vi "HEWH Get Rates.vi"(0 "Software Elapsed Time":T1 format="%<%H:%M:%S>t", 1 "Test Type - Rate":string(combo)="Rate", 5 "ANSI Rate in":T3, 9 "Gas Measurment Data":T2, 11 "error in (no error)":errorcluster, 12 "Gross Heating Value, Vol (Real, Dry)":dbl=1000.0 min=900.0 max=2600.0 step=1.0, 13 "CO CO2 Data Array":string[][](array[string])) -> (3 "ANSI Display 1":string, 4 "Rate Outputs":string[][](array[string]), 6 "Test Complete":bool, 10 "ANSI Rate out":T3, 14 "Raw Timer Output":T1 format="%<%H:%M:%S>t", 15 "error out":errorcluster)   [LabVIEW 2019]
uses:
  Range/Type Definitions/RANGE ANSI Rate.ctl
  Utility/Custom Pallet Controls/Custom Pallet Timer.ctl
  Drivers/Alicat Gas Meter Driver/Sub-VIs/Data Cluster.ctl
panel:
  # "Totalizer Timer"
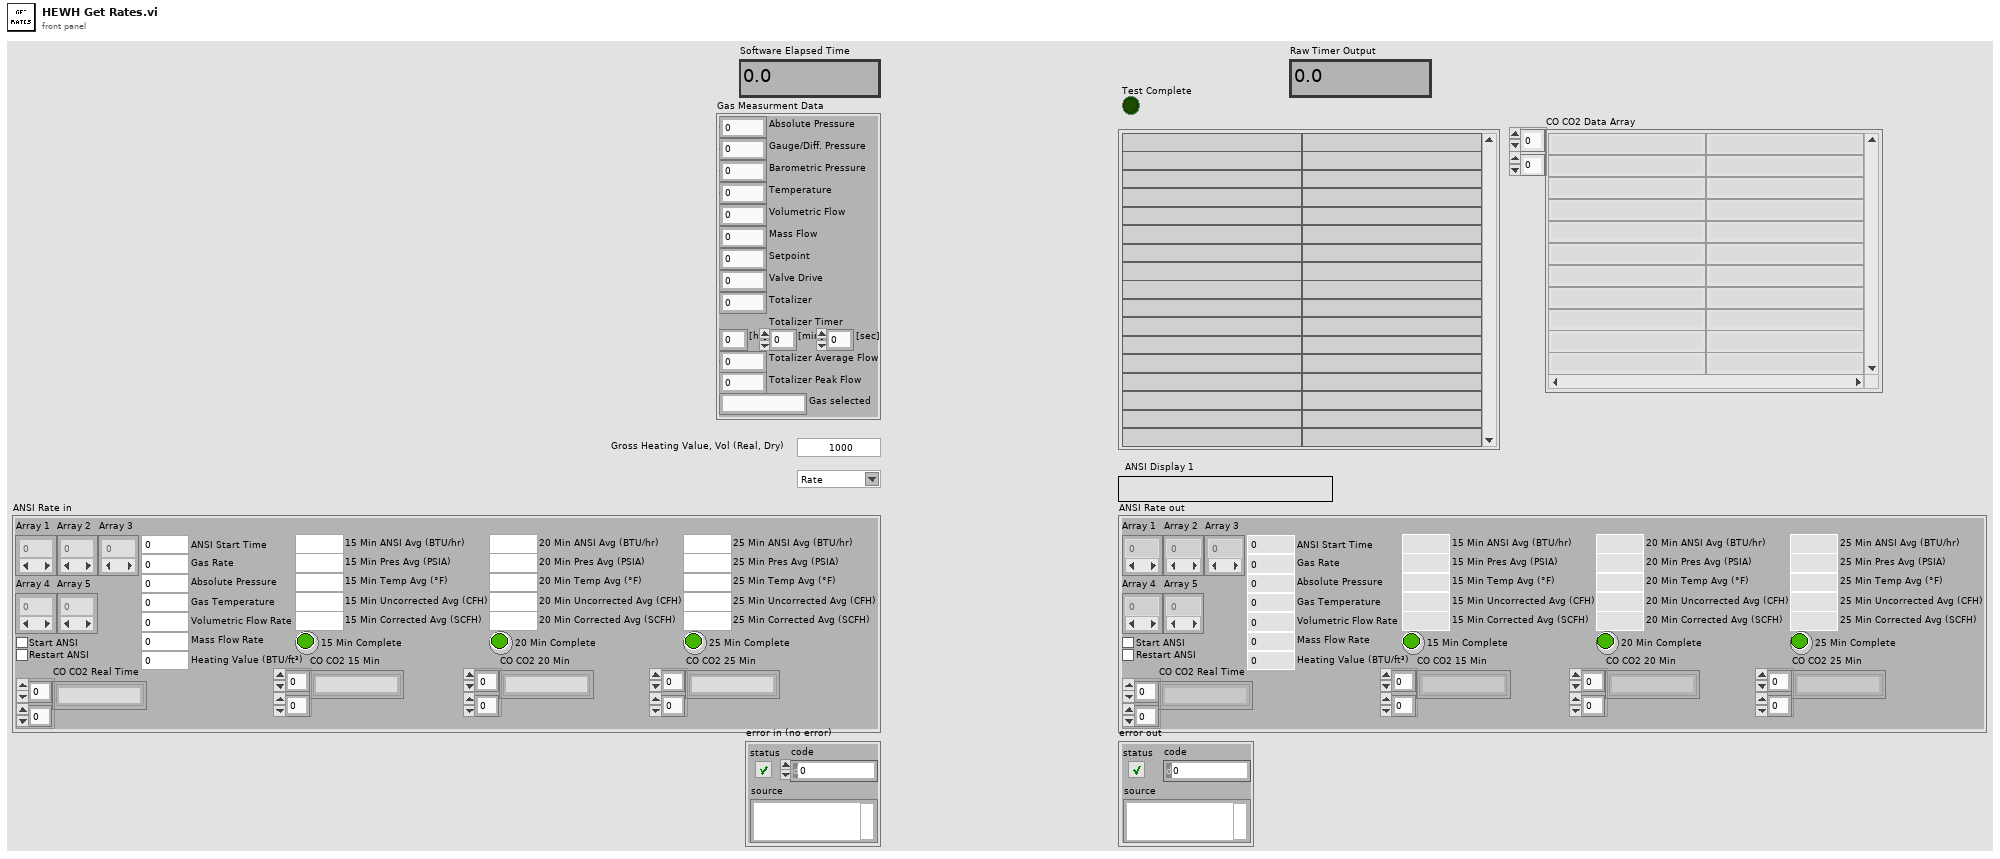
[diagram p1: front panel]
types:
  T1 = typedef "Custom Pallet Timer.ctl" = dbl
  T2 = typedef "Data Cluster.ctl" = cluster{"Absolute Pressure":dbl, "Gauge/Diff. Pressure":dbl, "Barometric Pressure":dbl, "Temperature":dbl, "Volumetric Flow":dbl, "Mass Flow":dbl, "Setpoint":dbl, "Valve Drive":dbl, "Totalizer":dbl, "[hr]":dbl, "[min]":dbl, "[sec]":dbl, "Totalizer Average Flow":dbl, "Totalizer Peak Flow":dbl, "Gas selected":string}
  T3 = typedef "RANGE ANSI Rate.ctl" = cluster{"Array 1":dbl[], "Array 3":dbl[], "Array 2":dbl[], "Start ANSI":bool, "ANSI Start Time":dbl, "Restart ANSI":bool, "15 Min ANSI Avg (BTU/hr)":dbl, "20 Min ANSI Avg (BTU/hr)":dbl, "25 Min ANSI Avg (BTU/hr)":dbl, "Absolute Pressure":dbl, "Gas Temperature":dbl, "Volumetric Flow Rate":dbl, "Mass Flow Rate":dbl, "Array 4":dbl[], "Array 5":dbl[], "Gas Rate":dbl, "15 Min Pres Avg (PSIA)":dbl, "20 Min Pres Avg (PSIA)":dbl, "25 Min Pres Avg (PSIA)":dbl, "15 Min Temp Avg (°F) ":dbl, "20 Min Temp Avg (°F)":dbl, "25 Min Temp Avg (°F)":dbl, "15 Min Uncorrected Avg (CFH)":dbl, "20 Min Uncorrected Avg (CFH)":dbl, "25 Min Uncorrected Avg (CFH)":dbl, "15 Min Corrected Avg (SCFH)":dbl, "20 Min Corrected Avg (SCFH)":dbl, "25 Min Corrected Avg (SCFH)":dbl, "15 Min Complete":bool, "20 Min Complete":bool, "25 Min Complete":bool, "Heating Value (BTU/ft³)":dbl, "CO CO2 15 Min":string[][], "CO CO2 20 Min":string[][], "CO CO2 25 Min":string[][], "CO CO2 Real Time":string[][]}
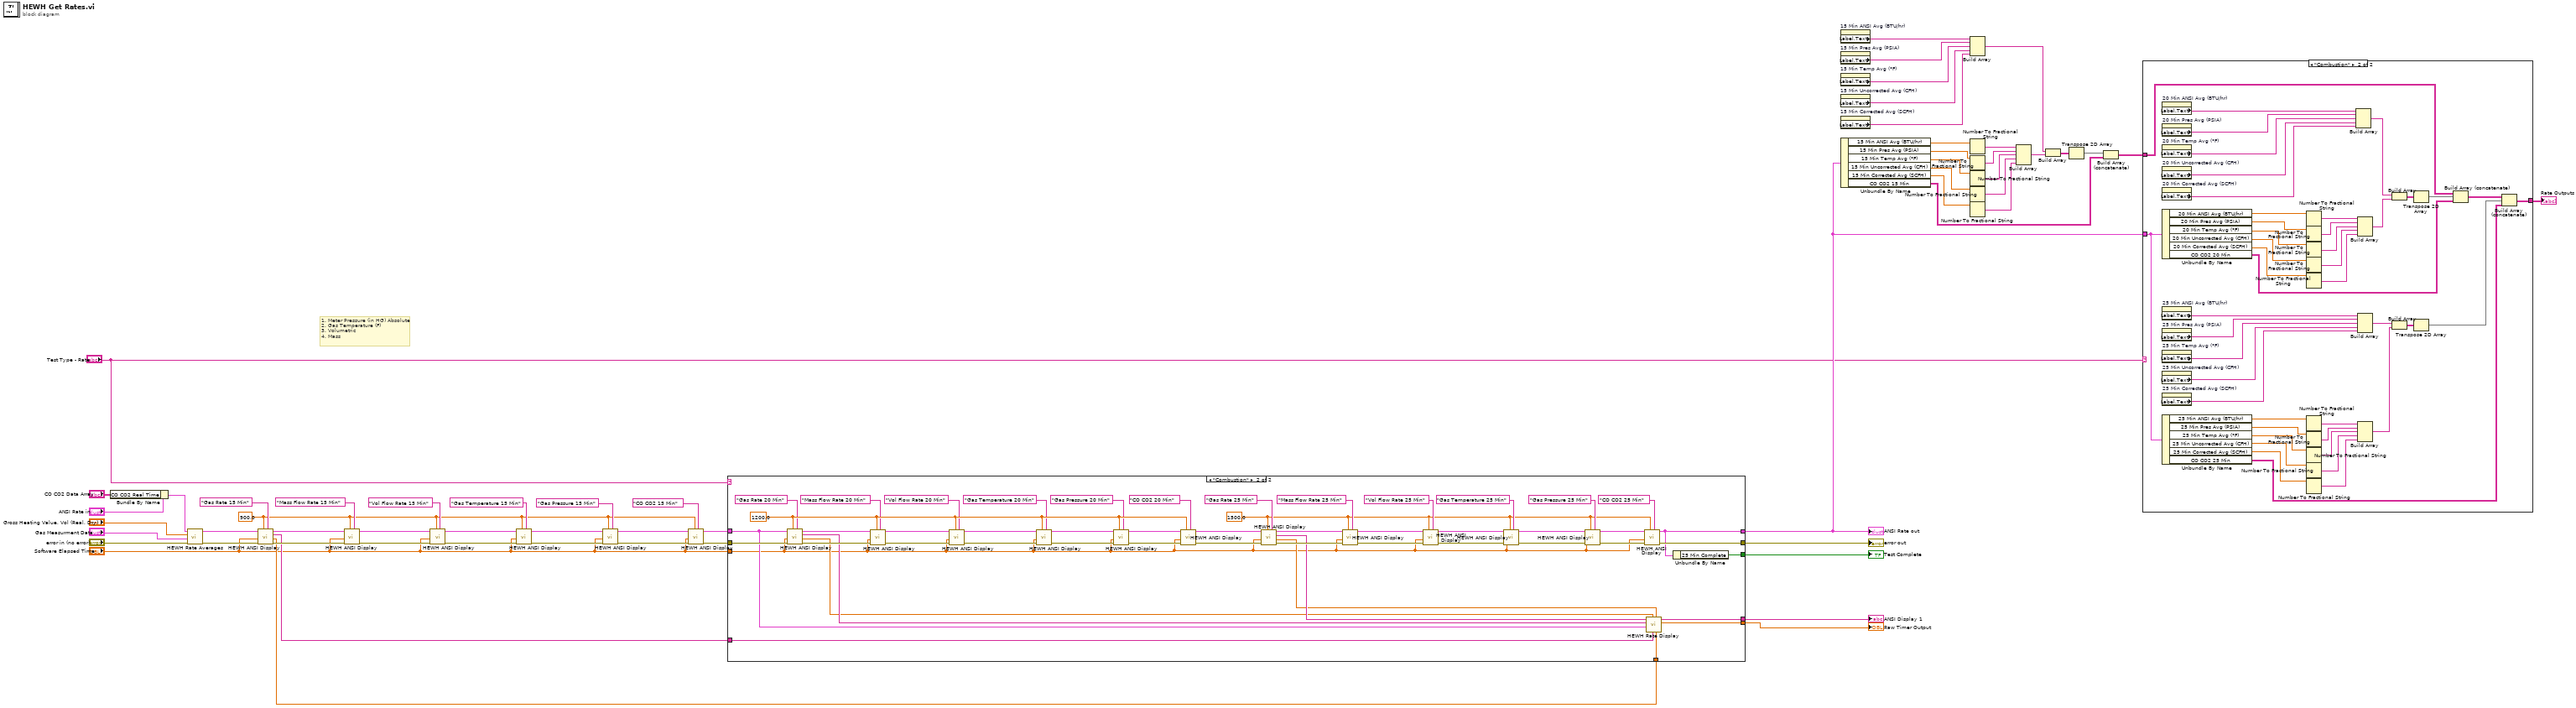
[diagram p0: block diagram]
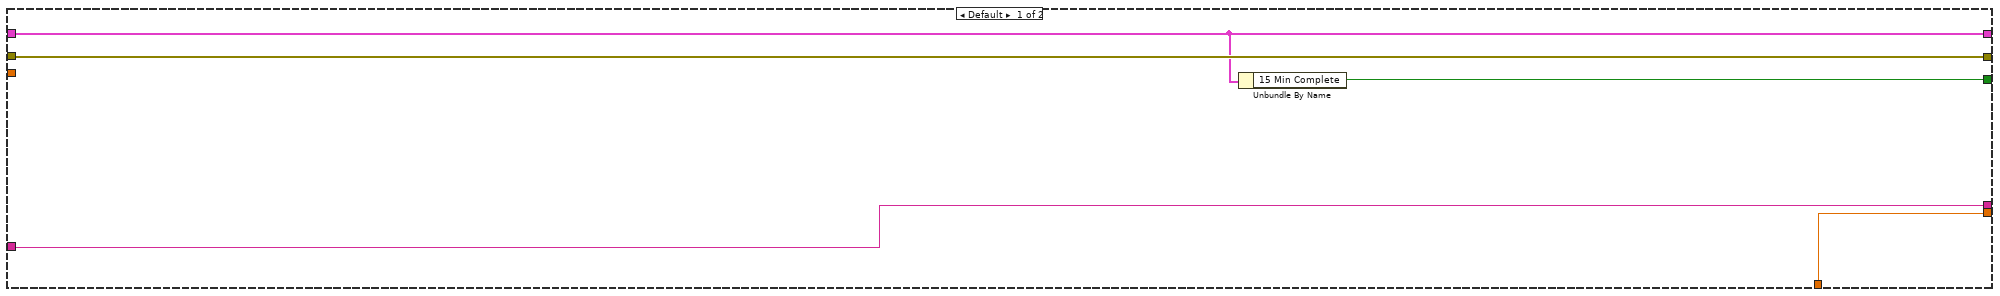
[diagram p3: hidden frame]
diagram:
  w8 = 900.0 ("Stop Timer")
  # "1. Meter Pressure (in HG) Absolute\n2. Gas Temperature (F)\n3. Volumetric\n4. Mass"
  n1 = Bundle By Name(cluster="ANSI Rate in", "CO CO2 Real Time"="CO CO2 Data Array") -> (w5:T3)
  n2 = call "HEWH Rate Averages.vi"("error in (no error)"="error in (no error)", "Gas Measurment Data"="Gas Measurment Data", "Gross Heating Value, Vol (Real, Dry)"="Gross Heating Value, Vol (Real, Dry)", "ANSI Rate in"=w5) -> ("error out"=w55:errorcluster, "ANSI Rate out"=w54:T3)  [unwired: 6 in]
  n3 = call "HEWH ANSI Display.vi"("Calculation Type"="Gas Rate 15 Min", "Stop Timer"=w8, "Error In"=w55, "Software Elapsed Time"="Software Elapsed Time", "ANSI Rate In"=w54) -> ("Error Out"=w49:errorcluster, "Raw Timer"=w20:dbl, "ANSI Display"=w22:string, "ANSI Rate Out"=w53:T3)  [unwired: 3 in]
  n4 = call "HEWH ANSI Display.vi"("Calculation Type"="Mass Flow Rate 15 Min", "Stop Timer"=w8, "Error In"=w49, "Software Elapsed Time"="Software Elapsed Time", "ANSI Rate In"=w53) -> ("Error Out"=w48:errorcluster, "ANSI Rate Out"=w52:T3)  [unwired: 3 in, 2 out]
  n5 = call "HEWH ANSI Display.vi"("Calculation Type"="Vol Flow Rate 15 Min", "Stop Timer"=w8, "Error In"=w48, "Software Elapsed Time"="Software Elapsed Time", "ANSI Rate In"=w52) -> ("Error Out"=w47:errorcluster, "ANSI Rate Out"=w51:T3)  [unwired: 3 in, 2 out]
  n6 = call "HEWH ANSI Display.vi"("Calculation Type"="Gas Temperature 15 Min", "Stop Timer"=w8, "Error In"=w47, "Software Elapsed Time"="Software Elapsed Time", "ANSI Rate In"=w51) -> ("Error Out"=w46:errorcluster, "ANSI Rate Out"=w50:T3)  [unwired: 3 in, 2 out]
  n7 = call "HEWH ANSI Display.vi"("Calculation Type"="Gas Pressure 15 Min", "Stop Timer"=w8, "Error In"=w46, "Software Elapsed Time"="Software Elapsed Time", "ANSI Rate In"=w50) -> ("Error Out"=w10:errorcluster, "ANSI Rate Out"=w12:T3)  [unwired: 3 in, 2 out]
  n8 = call "HEWH ANSI Display.vi"("Calculation Type"="CO CO2 15 Min", "Stop Timer"=w8, "Error In"=w10, "Software Elapsed Time"="Software Elapsed Time", "ANSI Rate In"=w12) -> ("Error Out"=w9:errorcluster, "ANSI Rate Out"=w11:T3)  [unwired: 3 in, 2 out]
  n9 = case shown="\"Combustion\"" "Test Type - Rate" {
    tunnel: w9 -> [w63 w113]
    tunnel: w11 -> [w62 w95]
    tunnel: [w63 w69] -> w45
    tunnel: [w62 w67] -> w44
    tunnel: "Software Elapsed Time" -> [_ w65]
    tunnel: [w61 w96] -> w23
    tunnel: w22 -> [w60 w94]
    tunnel: [w60 w93] -> w21
    tunnel: w20 -> [w59 w90]
    tunnel: [w59 w87] -> w19
    frame Default {
      n10 = Unbundle By Name(w62) -> ("15 Min Complete"=w61:bool)
    }
    frame "Combustion" {
      w66 = 1500.0 ("Stop Timer")
      w81 = 1200.0 ("Stop Timer")
      n11 = call "HEWH ANSI Display.vi"("Calculation Type"="Gas Rate 20 Min", "Stop Timer"=w81, "Error In"=w113, "Software Elapsed Time"=w65, "ANSI Rate In"=w95) -> ("Error Out"=w112:errorcluster, "Raw Timer"=w89:dbl, "ANSI Display"=w92:string, "ANSI Rate Out"=w105:T3)  [unwired: 3 in]
      n12 = call "HEWH ANSI Display.vi"("Calculation Type"="Mass Flow Rate 20 Min", "Stop Timer"=w81, "Error In"=w112, "Software Elapsed Time"=w65, "ANSI Rate In"=w105) -> ("Error Out"=w111:errorcluster, "ANSI Rate Out"=w106:T3)  [unwired: 3 in, 2 out]
      n13 = call "HEWH ANSI Display.vi"("Calculation Type"="Vol Flow Rate 20 Min", "Stop Timer"=w81, "Error In"=w111, "Software Elapsed Time"=w65, "ANSI Rate In"=w106) -> ("Error Out"=w110:errorcluster, "ANSI Rate Out"=w107:T3)  [unwired: 3 in, 2 out]
      n14 = call "HEWH ANSI Display.vi"("Calculation Type"="Gas Temperature 20 Min", "Stop Timer"=w81, "Error In"=w110, "Software Elapsed Time"=w65, "ANSI Rate In"=w107) -> ("Error Out"=w109:errorcluster, "ANSI Rate Out"=w108:T3)  [unwired: 3 in, 2 out]
      n15 = call "HEWH ANSI Display.vi"("Calculation Type"="Gas Pressure 20 Min", "Stop Timer"=w81, "Error In"=w109, "Software Elapsed Time"=w65, "ANSI Rate In"=w108) -> ("Error Out"=w83:errorcluster, "ANSI Rate Out"=w86:T3)  [unwired: 3 in, 2 out]
      n16 = call "HEWH ANSI Display.vi"("Calculation Type"="CO CO2 20 Min", "Stop Timer"=w81, "Error In"=w83, "Software Elapsed Time"=w65, "ANSI Rate In"=w86) -> ("Error Out"=w82:errorcluster, "ANSI Rate Out"=w85:T3)  [unwired: 3 in, 2 out]
      n17 = call "HEWH ANSI Display.vi"("Calculation Type"="Gas Rate 25 Min", "Stop Timer"=w66, "Error In"=w82, "Software Elapsed Time"=w65, "ANSI Rate In"=w85) -> ("Error Out"=w104:errorcluster, "Raw Timer"=w88:dbl, "ANSI Display"=w91:string, "ANSI Rate Out"=w100:T3)  [unwired: 3 in]
      n18 = call "HEWH ANSI Display.vi"("Calculation Type"="Mass Flow Rate 25 Min", "Stop Timer"=w66, "Error In"=w104, "Software Elapsed Time"=w65, "ANSI Rate In"=w100) -> ("Error Out"=w103:errorcluster, "ANSI Rate Out"=w99:T3)  [unwired: 3 in, 2 out]
      n19 = call "HEWH ANSI Display.vi"("Calculation Type"="Vol Flow Rate 25 Min", "Stop Timer"=w66, "Error In"=w103, "Software Elapsed Time"=w65, "ANSI Rate In"=w99) -> ("Error Out"=w102:errorcluster, "ANSI Rate Out"=w98:T3)  [unwired: 3 in, 2 out]
      n20 = call "HEWH ANSI Display.vi"("Calculation Type"="Gas Temperature 25 Min", "Stop Timer"=w66, "Error In"=w102, "Software Elapsed Time"=w65, "ANSI Rate In"=w98) -> ("Error Out"=w101:errorcluster, "ANSI Rate Out"=w97:T3)  [unwired: 3 in, 2 out]
      n21 = call "HEWH ANSI Display.vi"("Calculation Type"="Gas Pressure 25 Min", "Stop Timer"=w66, "Error In"=w101, "Software Elapsed Time"=w65, "ANSI Rate In"=w97) -> ("Error Out"=w70:errorcluster, "ANSI Rate Out"=w68:T3)  [unwired: 3 in, 2 out]
      n22 = call "HEWH ANSI Display.vi"("Calculation Type"="CO CO2 25 Min", "Stop Timer"=w66, "Error In"=w70, "Software Elapsed Time"=w65, "ANSI Rate In"=w68) -> ("Error Out"=w69:errorcluster, "ANSI Rate Out"=w67:T3)  [unwired: 3 in, 2 out]
      n23 = call "HEWH Rate Display.vi"("Raw Timer 15"=w90, "Raw Timer 25"=w88, "15 Min Display"=w94, "Raw Timer 20"=w89, "ANSI Rate Out"=w95, "20 Min Display"=w92, "25 Min Display"=w91) -> ("Raw Timer Output"=w87:T1, "Output Display"=w93:string)  [unwired: 2 in, 1 out]
      n24 = Unbundle By Name(w67) -> ("25 Min Complete"=w96:bool)
    }
  }
  "ANSI Display 1" <- w21
  "ANSI Rate out" <- w44
  "error out" <- w45
  "Test Complete" <- w23
  "Raw Timer Output" <- w19
  n25 = property on="15 Min ANSI Avg (BTU/hr)" class="DigNum (strict)"() -> ("Label.Text"=w31:string)  [unwired: 2 in, 2 out]
  n26 = property on="15 Min Pres Avg (PSIA)" class="DigNum (strict)"() -> ("Label.Text"=w30:string)  [unwired: 2 in, 2 out]
  n27 = property on="15 Min Temp Avg (°F)" class="DigNum (strict)"() -> ("Label.Text"=w29:string)  [unwired: 2 in, 2 out]
  n28 = property on="15 Min Uncorrected Avg (CFH)" class="DigNum (strict)"() -> ("Label.Text"=w28:string)  [unwired: 2 in, 2 out]
  n29 = property on="15 Min Corrected Avg (SCFH)" class="DigNum (strict)"() -> ("Label.Text"=w27:string)  [unwired: 2 in, 2 out]
  n30 = Unbundle By Name(w44) -> ("15 Min ANSI Avg (BTU/hr)"=w43:dbl, "15 Min Pres Avg (PSIA)"=w41:dbl, "15 Min Temp Avg (°F)"=w39:dbl, "15 Min Uncorrected Avg (CFH)"=w37:dbl, "15 Min Corrected Avg (SCFH)"=w35:dbl, "CO CO2 15 Min"=w1:string[][])
  n31 = Build Array(w31, w30, w29, w28, w27) -> (w26:string[])
  n32 = Number To Fractional String(number=w43) -> (F-format string=w42:string)  [unwired: 3 in]
  n33 = Number To Fractional String(number=w41) -> (F-format string=w40:string)  [unwired: 3 in]
  n34 = Number To Fractional String(number=w39) -> (F-format string=w38:string)  [unwired: 3 in]
  n35 = Number To Fractional String(number=w37) -> (F-format string=w36:string)  [unwired: 3 in]
  n36 = Number To Fractional String(number=w35) -> (F-format string=w34:string)  [unwired: 3 in]
  n37 = Build Array(w42, w40, w38, w36, w34) -> (w33:string[])
  n38 = Build Array(w26, w33) -> (w32:string[][])
  n39 = Transpose 2D Array(2D array=w32) -> (transposed array=w3:string[][])
  n40 = Build Array (concatenate)(w3, w1) -> (w2:string[][])
  n41 = case shown="\"Combustion\"" "Test Type - Rate" {
    tunnel: w44 -> [_ w158]
    tunnel: [w114 w117] -> w24
    tunnel: w2 -> [w114 w133]
    frame Default {
    }
    frame "Combustion" {
      n42 = property on="20 Min ANSI Avg (BTU/hr)" class="DigNum (strict)"() -> ("Label.Text"=w147:string)  [unwired: 2 in, 2 out]
      n43 = property on="20 Min Pres Avg (PSIA)" class="DigNum (strict)"() -> ("Label.Text"=w146:string)  [unwired: 2 in, 2 out]
      n44 = property on="20 Min Temp Avg (°F)" class="DigNum (strict)"() -> ("Label.Text"=w145:string)  [unwired: 2 in, 2 out]
      n45 = property on="20 Min Uncorrected Avg (CFH)" class="DigNum (strict)"() -> ("Label.Text"=w144:string)  [unwired: 2 in, 2 out]
      n46 = property on="20 Min Corrected Avg (SCFH)" class="DigNum (strict)"() -> ("Label.Text"=w143:string)  [unwired: 2 in, 2 out]
      n47 = Unbundle By Name(w158) -> ("20 Min ANSI Avg (BTU/hr)"=w157:dbl, "20 Min Pres Avg (PSIA)"=w156:dbl, "20 Min Temp Avg (°F)"=w155:dbl, "20 Min Uncorrected Avg (CFH)"=w154:dbl, "20 Min Corrected Avg (SCFH)"=w153:dbl, "CO CO2 20 Min"=w127:string[][])
      n48 = property on="25 Min ANSI Avg (BTU/hr)" class="DigNum (strict)"() -> ("Label.Text"=w126:string)  [unwired: 2 in, 2 out]
      n49 = property on="25 Min Pres Avg (PSIA)" class="DigNum (strict)"() -> ("Label.Text"=w125:string)  [unwired: 2 in, 2 out]
      n50 = property on="25 Min Temp Avg (°F)" class="DigNum (strict)"() -> ("Label.Text"=w124:string)  [unwired: 2 in, 2 out]
      n51 = property on="25 Min Uncorrected Avg (CFH)" class="DigNum (strict)"() -> ("Label.Text"=w123:string)  [unwired: 2 in, 2 out]
      n52 = property on="25 Min Corrected Avg (SCFH)" class="DigNum (strict)"() -> ("Label.Text"=w122:string)  [unwired: 2 in, 2 out]
      n53 = Unbundle By Name(w158) -> ("25 Min ANSI Avg (BTU/hr)"=w152:dbl, "25 Min Pres Avg (PSIA)"=w151:dbl, "25 Min Temp Avg (°F)"=w150:dbl, "25 Min Uncorrected Avg (CFH)"=w149:dbl, "25 Min Corrected Avg (SCFH)"=w148:dbl, "CO CO2 25 Min"=w115:string[][])
      n54 = Number To Fractional String(number=w157) -> (F-format string=w142:string)  [unwired: 3 in]
      n55 = Number To Fractional String(number=w156) -> (F-format string=w141:string)  [unwired: 3 in]
      n56 = Number To Fractional String(number=w155) -> (F-format string=w140:string)  [unwired: 3 in]
      n57 = Number To Fractional String(number=w154) -> (F-format string=w139:string)  [unwired: 3 in]
      n58 = Number To Fractional String(number=w153) -> (F-format string=w138:string)  [unwired: 3 in]
      n59 = Number To Fractional String(number=w152) -> (F-format string=w132:string)  [unwired: 3 in]
      n60 = Number To Fractional String(number=w151) -> (F-format string=w131:string)  [unwired: 3 in]
      n61 = Number To Fractional String(number=w150) -> (F-format string=w130:string)  [unwired: 3 in]
      n62 = Number To Fractional String(number=w149) -> (F-format string=w129:string)  [unwired: 3 in]
      n63 = Number To Fractional String(number=w148) -> (F-format string=w128:string)  [unwired: 3 in]
      n64 = Build Array(w147, w146, w145, w144, w143) -> (w136:string[])
      n65 = Build Array(w142, w141, w140, w139, w138) -> (w135:string[])
      n66 = Build Array(w126, w125, w124, w123, w122) -> (w120:string[])
      n67 = Build Array(w132, w131, w130, w129, w128) -> (w119:string[])
      n68 = Build Array(w136, w135) -> (w137:string[][])
      n69 = Build Array(w120, w119) -> (w121:string[][])
      n70 = Transpose 2D Array(2D array=w137) -> (transposed array=w134:string[][])
      n71 = Transpose 2D Array(2D array=w121) -> (transposed array=w116:string[][])
      n72 = Build Array (concatenate)(w133, w134, w127) -> (w118:string[][])
      n73 = Build Array (concatenate)(w118, w116, w115) -> (w117:string[][])
    }
  }
  "Rate Outputs" <- w24
